vi "ISMBUS_InitPort.vi"(0 "Module":T1, 5 "ComPort":i32, 11 "Fehler (Eingang - kein Fehler)":errorcluster) -> (15 "Fehler (Ausgang)":errorcluster)   [LabVIEW 2016]
uses:
  ISMBUS_Module.ctl
  ISMBUS_Channel.ctl
  ISMBUS32.DLL
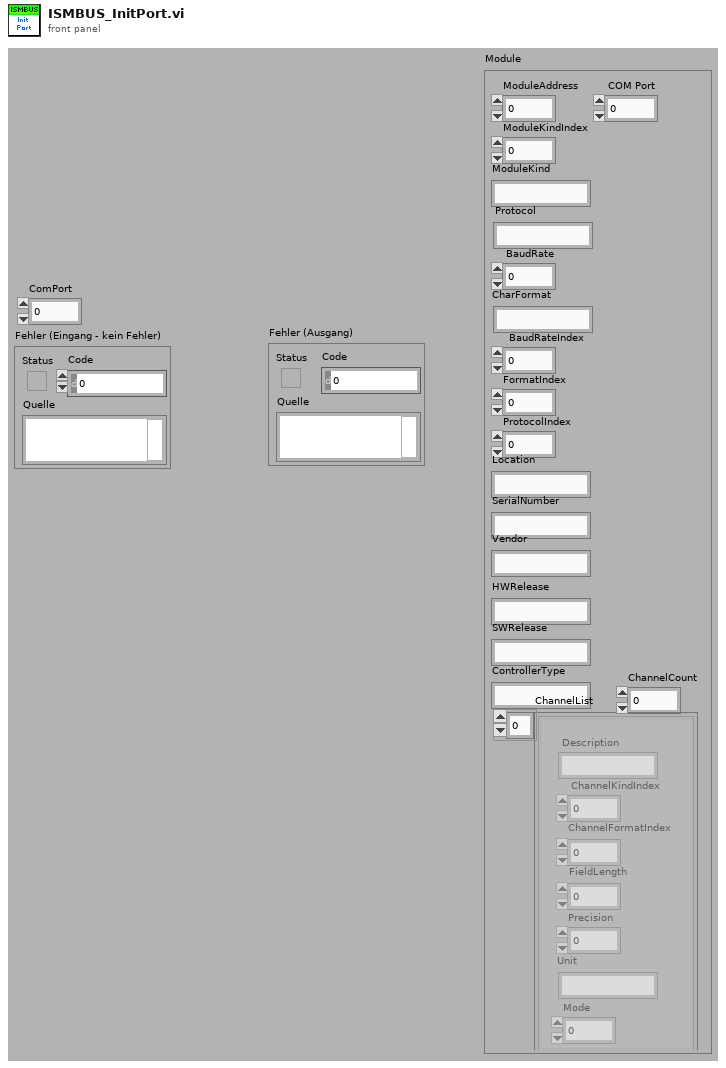
[diagram p1: front panel]
types:
  T1 = typedef "ISMBUS_Module.ctl" = cluster{"ModuleAddress":i32, "ModuleKindIndex":i32, "ModuleKind":string, " Protocol":string, " BaudRate":i32, "CharFormat":string, "BaudRateIndex":i32, "FormatIndex":i32, "ProtocolIndex":i32, "Location":string, "SerialNumber":string, "Vendor":string, "HWRelease":string, "SWRelease":string, "ControllerType":string, "ChannelList":T2[], "ChannelCount":i32, " COM Port":i32}
  T2 = typedef "ISMBUS_Channel.ctl" = cluster{" Description":string, " ChannelKindIndex":i32, "ChannelFormatIndex":i32, " FieldLength":i32, "Precision":i32, "Unit":string, "Mode":i32}
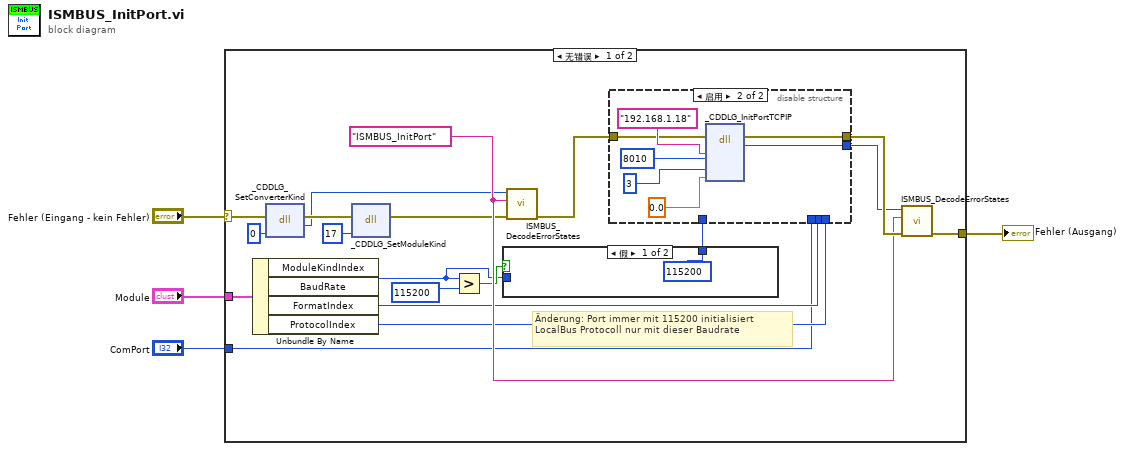
[diagram p0: block diagram]
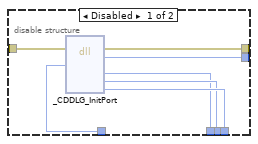
[diagram p2: hidden frame]
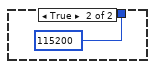
[diagram p3: hidden frame]
diagram:
  n1 = case shown="无错误" "Fehler (Eingang - kein Fehler)" {
    selector: "Fehler (Eingang - kein Fehler)" -> [w20 w40]
    tunnel: [w22 w40] -> w3
    tunnel: "Module" -> [w16 _]
    tunnel: "ComPort" -> [w10 _]
    frame No Error {
      w19 = "ISMBUS_InitPort" ("Location")
      # "Änderung: Port immer mit 115200 initialisiert\nLocalBus Protocoll nur mit dieser Baudrate"
      n2 = Unbundle By Name(w16) -> ("BaudRate"=w6:i32, "FormatIndex"=w11:i32, "ProtocolIndex"=w14:i32)  [unwired: 1 out]
      n3 = dll-call lib="ISMBUS32.DLL" fn="_CDDLG_SetConverterKind"(error in=w20, "ConverterKind"=0) -> (error out=w15:errorcluster, "Rückgabetyp"=w12:i32)  [unwired: 3 in, 1 out]
      n4 = dll-call lib="ISMBUS32.DLL" fn="_CDDLG_SetModuleKind"(error in=w15, "Modulekind"=17) -> (error out=w13:errorcluster)  [unwired: 3 in, 2 out]
      n5 = Greater?(x=w6, y=115200) -> (0:w8:bool)
      n6 = case shown="假" w8 {
        tunnel: [115200 ("y") 115200 ("y")] -> w7
        tunnel: w6 -> [_ _]
        frame False {
        }
        frame True {
        }
      }
      n7 = call "ISMBUS_DecodeErrorStates.vi"("Fehler (Eingang - kein Fehler)"=w13, "Location"=w19, "ISMBUS_Error State"=w12) -> ("Fehler (Ausgang)"=w18:errorcluster)  [unwired: 8 out]
      n8 = disable-structure shown="启用" {
        disable-tunnel: [w30 w32] -> w23
        disable-tunnel: [w29 w33] -> w21
        disable-tunnel: w18 -> [w28 w31]
        disable-tunnel: w14 -> [w27 _]
        disable-tunnel: w11 -> [w26 _]
        disable-tunnel: w10 -> [w25 _]
        disable-tunnel: w7 -> [w24 _]
        frame Disabled {
          n9 = dll-call lib="ISMBUS32.DLL" fn="_CDDLG_InitPort"(error in=w28, "BaudRate"=w24, "ComPort"=w25, "Format"=w26, "Protocol"=w27) -> (error out=w30:errorcluster, "Rückgabetyp"=w29:i32)  [unwired: 6 in, 1 out]
        }
        frame Enabled {
          n10 = dll-call lib="ISMBUS32.DLL" fn="_CDDLG_InitPortTCPIP"(error in=w31, "IPAddr"="192.168.1.18", "IPPort"=8010, "Prot"=3, "TimeoutS"=0.0) -> (error out=w32:errorcluster, "Rückgabetyp"=w33:i32)  [unwired: 6 in, 1 out]
        }
      }
      n11 = call "ISMBUS_DecodeErrorStates.vi"("Fehler (Eingang - kein Fehler)"=w23, "Location"=w19, "ISMBUS_Error State"=w21) -> ("Fehler (Ausgang)"=w22:errorcluster)  [unwired: 8 out]
    }
    frame Error {
    }
  }
  "Fehler (Ausgang)" <- w3
